vi "Generate Assert VI Template Path.vi"(8 "error in (no error)":errorcluster, 9 "Operation":string, 10 "Data Type":T1) -> (0 "error out":errorcluster, 2 "Template Path":path)   [LabVIEW 2016]
uses:
  <vilib>/Utility/Data Type/Type Definitions/Data Type.ctl
  <vilib>/Utility/Data Type/NI_Data Type.lvlib
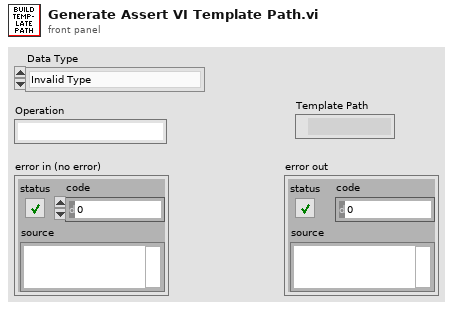
[diagram p1: front panel]
types:
  T1 = typedef "NI_Data Type.lvlib/Data Type.ctl" = enum8{"Invalid Type", "Void", "I8", "I16", "I32", "I64", "U8", "U16", "U32", "U64", "Single Float", "Double Float", "Extended Float", "Single Complex", "Double Complex", "Extended Complex", "Enum U8", "Enum U16", "Enum U32", "Enum U64", "Single Float With Unit", "Double Float With Unit", "Extended Float With Unit", "Single Complex with Unit", "Double Complex with Unit", "Extended Complex with Unit", "Boolean", "String", "Path", "Picture", "Tag", "Array", "Cluster", "Variant", "LV Variant", "Waveform", "Timestamp", "Digital Waveform", "Digital Data", "ExpressData", "Refnum", "External Data", "VI", "Poly VI", "LabVIEW Class Instance", "Fixed Point"}
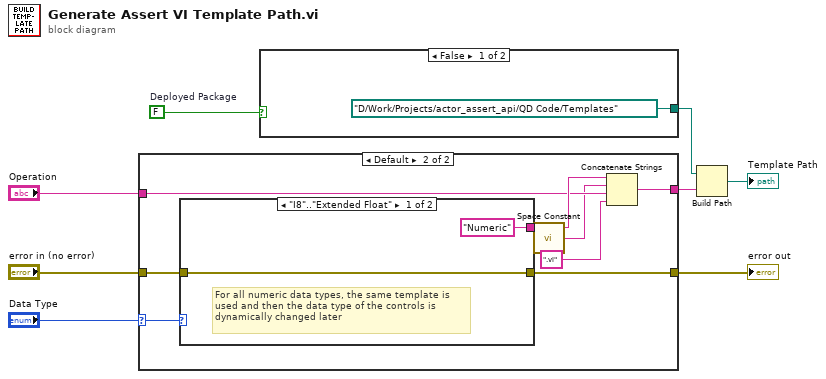
[diagram p0: block diagram]
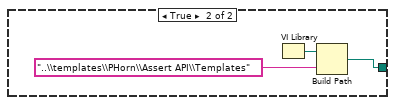
[diagram p2: hidden frame]
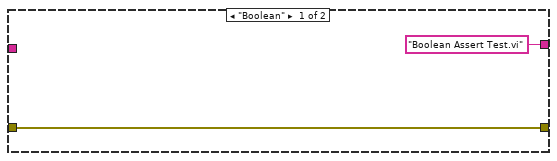
[diagram p3: hidden frame]
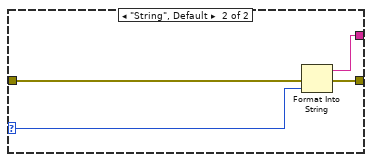
[diagram p4: hidden frame]
diagram:
  w1 = FALSE  # Deployed Package
  n1 = case shown="Default" "Data Type" {
    selector: "Data Type" -> [_ w16]
    tunnel: [w9 w18] -> w8
    tunnel: "error in (no error)" -> [w9 w17]
    tunnel: "Operation" -> [_ w13]
    tunnel: ["Boolean Assert Test.vi" w11] -> w2
    frame "Boolean" {
    }
    frame Default {
      n2 = case shown="\"I8\"..\"Extended Float\"" w16 {
        selector: w16 -> [_ w22]
        tunnel: [w19 w24] -> w18
        tunnel: w17 -> [w19 w23]
        tunnel: ["Numeric" w21] -> w15
        frame "I8".."Extended Float" {
          # "For all numeric data types, the same template is used and then the data type of the controls is dynamically changed later"
        }
        frame "String", Default {
          n3 = Format Into String(error in=w23, w22) -> (resulting string=w21:string, error out=w24:errorcluster)  [unwired: 2 in]
        }
      }
      n4 = call <vilib>:"Space Constant.vi"() -> ("String"=w12:string)
      n5 = Concatenate Strings(w15, w12, w13, ".vi") -> (w11:string)
    }
  }
  "error out" <- w8
  n6 = case shown="False" w1 {
    tunnel: [path "D:/Work/Projects/actor_assert_api/QD Code/Templates" ("template") w28] -> w4
    frame False {
    }
    frame True {
      n7 = VI Library() -> (path=w27:path)
      n8 = Build Path(base path=w27, name or relative path="..\\templates\\PHorn\\Assert API\\Templates") -> (appended path=w28:path)
    }
  }
  n9 = Build Path(base path=w4, name or relative path=w2) -> (appended path=→"Template Path":path)
